vi "Vision_Aim.vi"(0 "Cam_Angle":dbl=5.106668854486864, 1 "Yaw":dbl=9.462154437498084, 2 "Auto_Aim":bool, 3 "Auto_Shoot_Aim":bool, 6 "Hunt":bool) -> (5 "Aimed?":bool, 7 "Auto_Aim_Enable":bool, 8 "Enable_Cam":bool, 9 "Set_Point":dbl, 10 "CAM_Reset_IMU":bool)   [LabVIEW 2015]
uses:
  <vilib>/Rock Robotics/Network Tables/NT Read Number.vi
  <vilib>/Rock Robotics/Network Tables/NT Read Boolean.vi
  Global_Var/Drive_Global.vi
panel:
  out "Boolean":bool
  in  "Turning_Extra":dbl=30.0
  in  "Error_Delta":dbl=0.5
  out "Waveform Chart 2":cluster{i16, i16, i16}(graph)={0, 1, 0}
  out "Waveform Chart":cluster{"Cam_Angle":dbl, "Output":dbl}(graph)
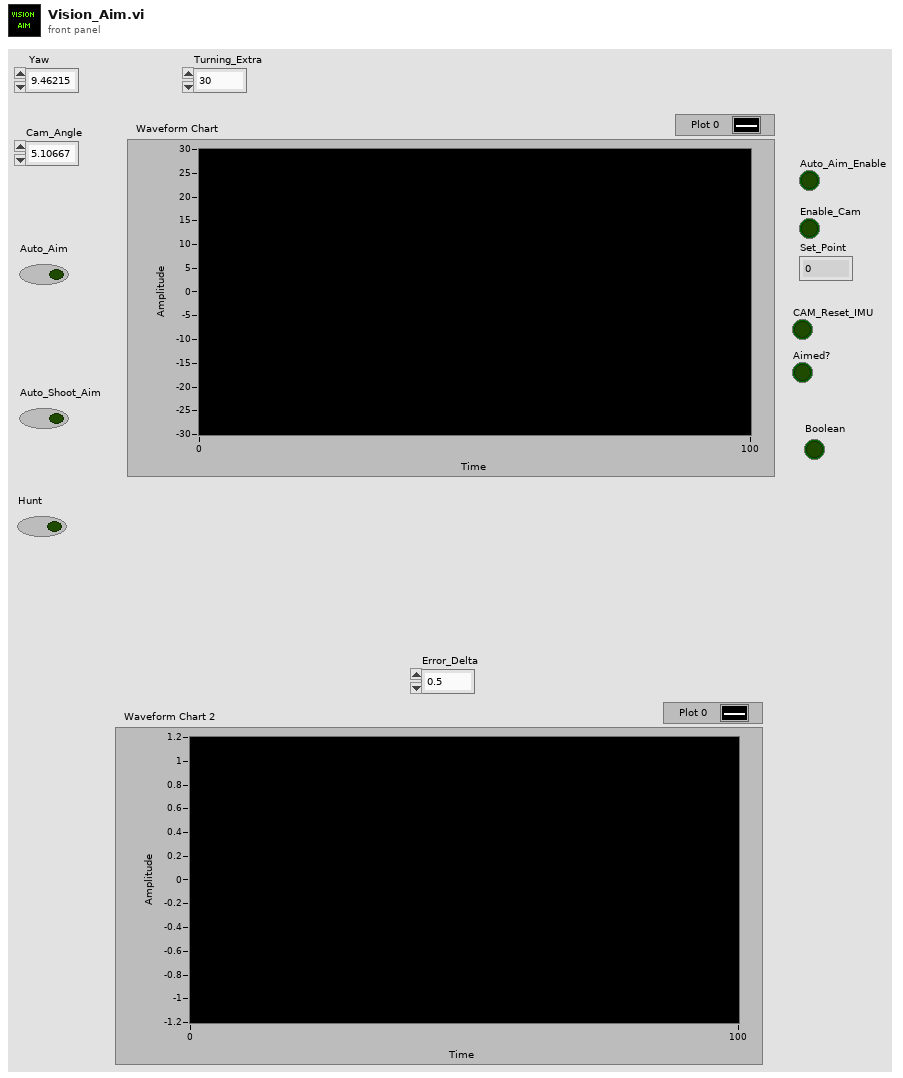
[diagram p1: front panel]
types:
  T1 = enum16{"Rising", "Falling", "Falling and Rising"}
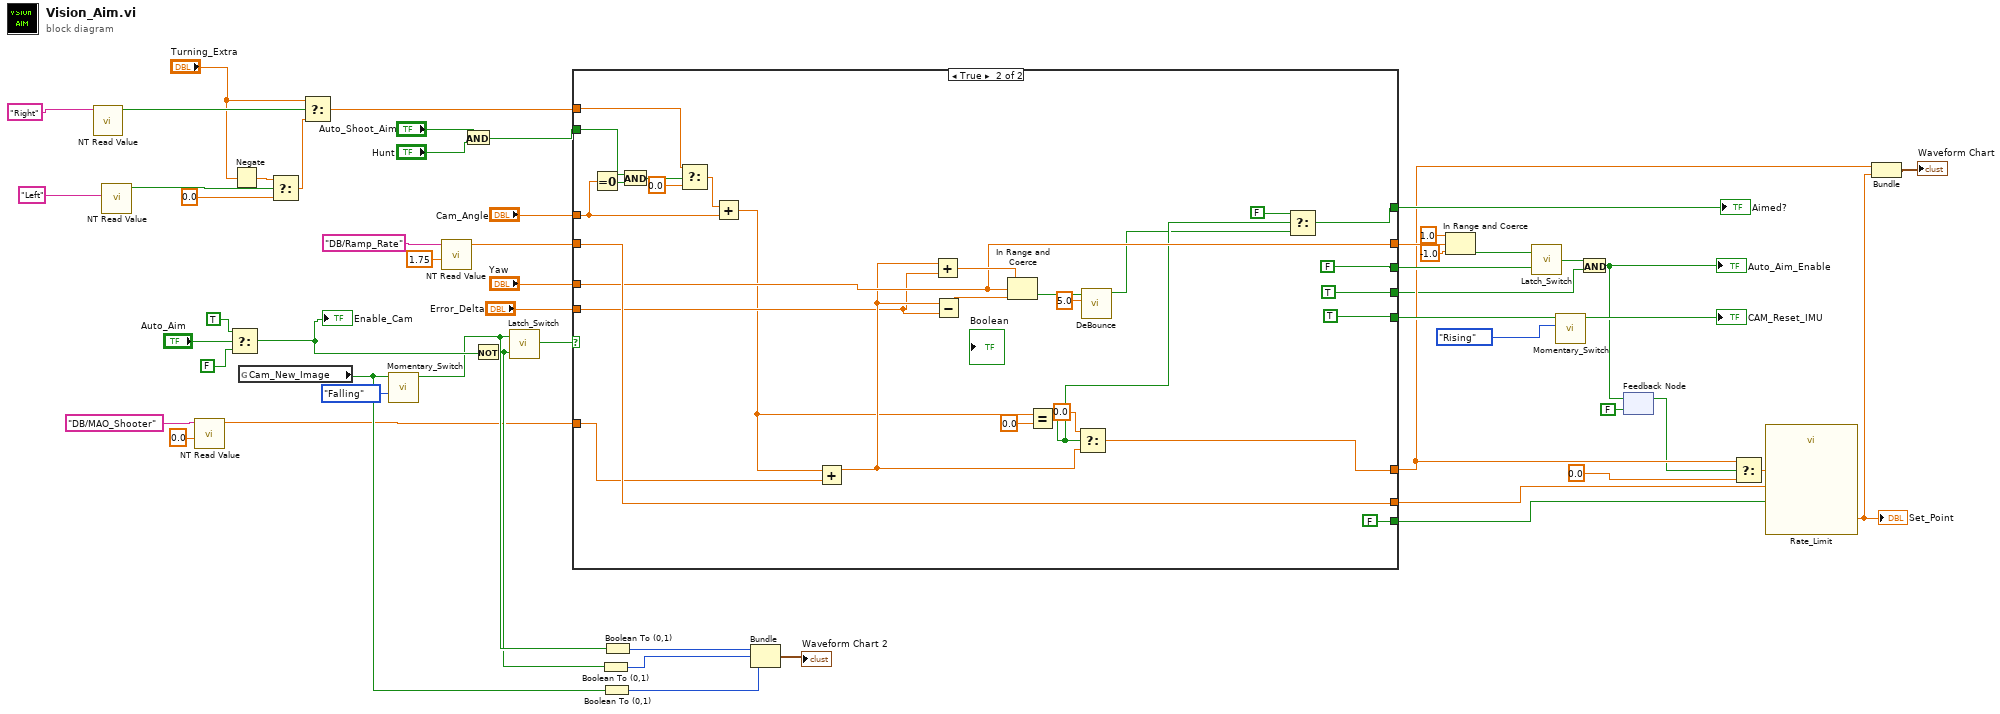
[diagram p0: block diagram]
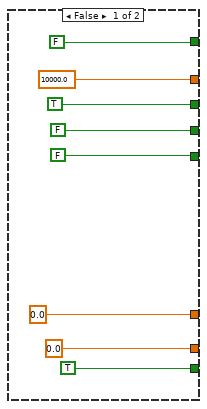
[diagram p2: hidden frame]
diagram:
  n1 = call-poly <vilib>:"NT Read Value.vi"("Name"="Right" ("refnum name")) -> ("Boolean"=w11:bool)  [unwired: 9 in, 1 out]
  n2 = call-poly <vilib>:"NT Read Value.vi"("Name"="Left" ("refnum name")) -> ("Boolean"=w12:bool)  [unwired: 9 in, 1 out]
  n3 = call-poly <vilib>:"NT Read Value.vi"("Default Value"=0.0, "Name"="DB/MAO_Shooter" ("refnum name")) -> ("Numeric"=w18:dbl)  [unwired: 8 in, 1 out]
  n4 = Select(t=TRUE, s="Auto_Aim", f=FALSE) -> (s? t:f=w41:bool)
  "Enable_Cam" <- w41
  n5 = Negate(x="Turning_Extra") -> (-x=w8:dbl)
  n6 = global read "Drive_Global.vi" "Cam_New_Image"() -> (w34:bool)
  n7 = Select(t=w8, s=w12, f=0.0) -> (s? t:f=w10:dbl)
  n8 = Select(t="Turning_Extra", s=w11, f=w10) -> (s? t:f=w6:dbl)
  n9 = call "Momentary_Switch.vi"("Type"=T1."Falling", "input_bol"=w34) -> ("out"=w39:bool)  [unwired: 9 in]
  n10 = call-poly <vilib>:"NT Read Value.vi"("Default Value"=1.75, "Name"="DB/Ramp_Rate" ("refnum name")) -> ("Numeric"=w14:dbl)  [unwired: 8 in, 1 out]
  n11 = And(x="Auto_Shoot_Aim", y="Hunt") -> (x .and. y?=w1:bool)
  n12 = Not(x=w41) -> (.not. x?=w38:bool)
  n13 = call "Latch_Switch.vi"("Reset"=w38, "In"=w39) -> ("Out"=w40:bool)
  n14 = case shown="True" w40 {
    tunnel: [0.0 ("Cam_Angle") w80] -> w26
    tunnel: [0.0 w91] -> w50
    tunnel: "Cam_Angle" -> [_ w68]
    tunnel: [FALSE TRUE] -> w21
    tunnel: w14 -> [_ w91]
    tunnel: [FALSE TRUE] -> w53
    tunnel: "Yaw" -> [_ w79]
    tunnel: [FALSE w74] -> w51
    tunnel: w18 -> [_ w78]
    tunnel: [TRUE FALSE] -> w49
    tunnel: [10000.0 ("Yaw") w79] -> w32
    tunnel: [TRUE FALSE] -> w29
    tunnel: "Error_Delta" -> [_ w76]
    tunnel: w1 -> [_ w65]
    tunnel: w6 -> [_ w64]
    frame False {
    }
    frame True {
      n15 = Equal To 0?(x=w68) -> (x = 0?=w67:bool)
      n16 = And(x=w65, y=w67) -> (x .and. y?=w66:bool)
      n17 = Select(t=w64, s=w66, f=0.0) -> (s? t:f=w69:dbl)
      n18 = Add(x=w69, y=w68) -> (x+y=w71:dbl)
      n19 = Add(x=w71, y=w78) -> (x+y=w77:dbl)
      n20 = Add(x=w77, y=w76) -> (x+y=w89:dbl)
      n21 = Subtract(x=w77, y=w76) -> (x-y=w88:dbl)
      n22 = In Range and Coerce(upper limit=w89, x=w79, lower limit=w88) -> (In Range?=w87:bool)  [unwired: 1 out]
      n23 = Equal?(x=w71, y=0.0) -> (x = y?=w75:bool)
      n24 = Select(t=0.0, s=w75, f=w77) -> (s? t:f=w80:dbl)
      n25 = call "DeBounce.vi"("DB_Count"=5.0, "Value"=w87) -> ("BD_Value"=w72:bool)  [unwired: 9 in]
      n26 = Select(t=FALSE, s=w75, f=w72) -> (s? t:f=w74:bool)
    }
  }
  "Aimed?" <- w51
  n27 = Boolean To (0,1)(Boolean=w38) -> (0, 1=w36:i16)
  n28 = Boolean To (0,1)(Boolean=w34) -> (0, 1=w33:i16)
  n29 = Boolean To (0,1)(Boolean=w39) -> (0, 1=w37:i16)
  n30 = Bundle(w37, w36, w33) -> (→"Waveform Chart 2":cluster{i16, i16, i16})  [unwired: 1 in]
  n31 = In Range and Coerce(upper limit=1.0, x=w32, lower limit=-1.0) -> (In Range?=w24:bool)  [unwired: 1 out]
  n32 = call "Latch_Switch.vi"("Reset"=w29, "In"=w24) -> ("Out"=w28:bool)
  n33 = call "Momentary_Switch.vi"("Type"=T1."Rising", "input_bol"=w53) -> ("out"=→"CAM_Reset_IMU":bool)  [unwired: 9 in]
  n34 = And(x=w28, y=w21) -> (x .and. y?=w20:bool)
  "Auto_Aim_Enable" <- w20
  n35 = feedback-in #1(w20) -> ()
  n36 = feedback #1(FALSE) -> (w23:bool)
  n37 = Select(t=w26, s=w23, f=0.0) -> (s? t:f=w27:dbl)
  n38 = call "Rate_Limit.vi"("Reset"=w49, "Ramp_Rate"=w50, "Input"=w27) -> ("Output"=w47:dbl)  [unwired: 8 in]
  "Set_Point" <- w47
  n39 = Bundle("t"=w26, "Output"=w47) -> (→"Waveform Chart":cluster{"t":dbl, "Output":dbl})  [unwired: 1 in]
